vi "CTRE_Phoenix_TalonSRX_Open.vi"(6 "Invert":bool, 8 "error in":errorcluster, 10 "Device Number":u8) -> (0 "error out":errorcluster, 3 "CAN Talon SRX Ref":T1={"DeviceStatus"={"status"=FALSE, "code"=0, "source"=""}, "Type"=enum."PWM", "PWM"={"PWM Channel"=enum."PWM 1", "DeadBand"={"Name"="", "maxPositivePwm"=0, "minPositivePwm"=0, "centerPwm"=0, "maxNegativePwm"=0, "minNegativePwm"=0, "angularRange"=0}}, "CAN"={"Device Number"=0, "SetOutput VI Ref"=variant(enum8{"Percent VBus", "Current", "Speed", "Position", "Voltage"} enum."Percent VBus"), "GetOutput VI Ref"=variant(refnum<k1> refnum), "Enable VI Ref"=variant(dbl 12.0), "Disable VI Ref"=variant(enum8{"Percent VBus", "Speed", "Position", "Slave", "Unchanged / Invalid", "Voltage Compensation", "Current", "Motion Profile"} enum."Percent VBus"), "Data"=variant}, "Invert"=FALSE, "DIO PWM"={"PWM \"Enable\" Channel"=enum."Invalid", "DIOChannel"=enum."Invalid", "PWM Rate"=0.0}})   [LabVIEW 2020]
doc: "Creates a reference to the CAN-connected Talon SRX motor controller you specify. You must open a reference before using any other VIs on this palette. After you open a reference to the Talon SRX motor controller, you can use the other Talon SRX VIs to configure and control the Talon SRX. This reference is compatible with the WPI Robotics Motor VIs.\n\n<B>Control Mode</B> is the desired control mode of the Talon SRX.\n\n<B>Device Number</B> is the Talon SRX Device ID on the CAN bus.\n\n<B>Master Device Number</B> is the CAN bus Device ID of the master controller that this controller is to follow.\n\n<B>Invert</B> enables/disables inverting the motor when using the WPI Robotics SetOutput.vi."
uses:
  <vilib>/Rock Robotics/WPI/MotorControl/WPI_MotorControlDeviceRef.ctl
  <vilib>/Rock Robotics/WPI/MotorControl/WPI_MotorControlType.ctl
  <vilib>/Rock Robotics/SystemInterfaces/DIO/FPGA_DIOPWMChannel.ctl
  <vilib>/Rock Robotics/WPI/PWM/WPI_PWMDeadband.ctl
  <vilib>/Rock Robotics/SystemInterfaces/DIO/FPGA_DIOChannel.ctl
  <vilib>/Rock Robotics/WPI/ThirdParty/Phoenix-LabVIEW/Motor Controller/Controls/CTRE_Phoenix_MotorControl_DevRefData.ctl
  <vilib>/Rock Robotics/WPI/ThirdParty/Phoenix-LabVIEW/Motor Controller/Controls/CTRE_Phoenix_MotorControl_ControlMode.ctl
  <vilib>/Rock Robotics/WPI/ThirdParty/Phoenix-LabVIEW/Controls/DriverLib.ctl
  <vilib>/Rock Robotics/SystemInterfaces/NetworkCommunication/NetComm_UsageReport_ResourceType.ctl
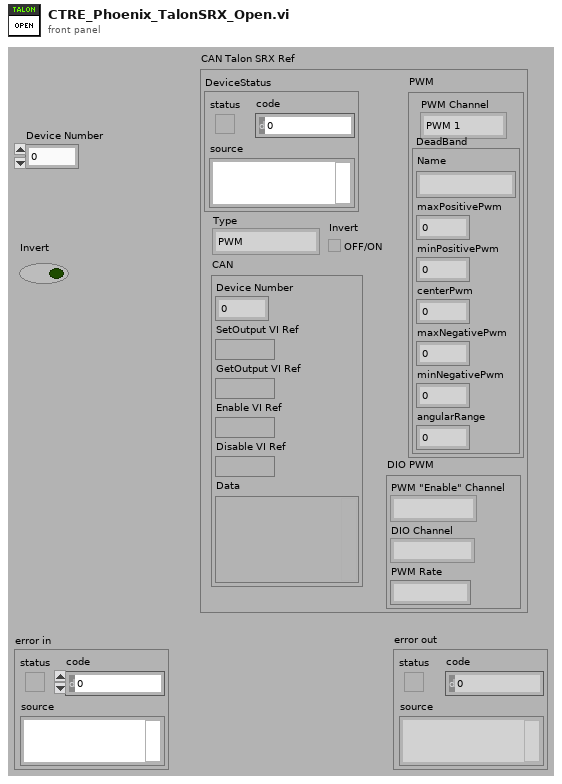
[diagram p1: front panel]
types:
  T1 = typedef "WPI_MotorControlDeviceRef.ctl" = cluster{"DeviceStatus":errorcluster, "Type":T2, "PWM":cluster{"PWM Channel":T3, "DeadBand":T4}, "CAN":cluster{"Device Number":u8, "SetOutput VI Ref":variant, "GetOutput VI Ref":variant, "Enable VI Ref":variant, "Disable VI Ref":variant, "Data":variant}, "Invert":bool, "DIO PWM":cluster{"PWM \"Enable\" Channel":T3, "DIOChannel":T5, "PWM Rate":dbl}}
  T2 = typedef "WPI_MotorControlType.ctl" = enum16{"PWM", "CAN", "DIO PWM"}
  T3 = typedef "FPGA_DIOPWMChannel.ctl" = enum8{"PWM 0", "PWM 1", "PWM 2", "PWM 3", "PWM 4", "PWM 5", "PWM 6", "PWM 7", "PWM 8", "PWM 9", "PWM MXP 0", "PWM MXP 1", "PWM MXP 2", "PWM MXP 3", "PWM MXP 4", "PWM MXP 5", "PWM MXP 6", "PWM MXP 7", "PWM MXP 8", "PWM MXP 9", "Invalid"}
  T4 = typedef "WPI_PWMDeadband.ctl" = cluster{"Name":string, "maxPositivePwm":i32, "minPositivePwm":i32, "centerPwm":i32, "maxNegativePwm":i32, "minNegativePwm":i32, "angularRange":u16}
  T5 = typedef "FPGA_DIOChannel.ctl" = enum8{"DIO 0", "DIO 1", "DIO 2", "DIO 3", "DIO 4", "DIO 5", "DIO 6", "DIO 7", "DIO 8", "DIO 9", "DIO MXP 0", "DIO MXP 1", "DIO MXP 2", "DIO MXP 3", "DIO MXP 4", "DIO MXP 5", "DIO MXP 6", "DIO MXP 7", "DIO MXP 8", "DIO MXP 9", "DIO MXP 10", "DIO MXP 11", "DIO MXP 12", "DIO MXP 13", "DIO MXP 14", "DIO MXP 15", "SPI Port CS1", "SPI Port CS2", "SPI Port CS3", "SPI Port MISO", "SPI Port MOSI", "Invalid"}
  T6 = typedef "CTRE_Phoenix_MotorControl_DevRefData.ctl" = cluster{"Library":path, "handle":u64, "Control Mode":T7, "UsageFrame":u32, "RefNumName":string, "arbID":u32}
  T7 = typedef "CTRE_Phoenix_MotorControl_ControlMode.ctl" = u16
  T8 = typedef "NetComm_UsageReport_ResourceType.ctl" = enum8{"Controller", "Module", "Language", "CANPlugin", "Accelerometer", "ADXL345", "AnalogChannel", "AnalogTrigger", "AnalogTriggerOutput", "CANJaguar", "Compressor", "Counter", "Dashboard", "DigitalInput", "DigitalOutput", "DriverStationCIO", "DriverStationEIO", "DriverStationLCD", "Encoder", "GearTooth", "Gyro", "I2C", "Framework", "Jaguar", "Joystick", "Kinect", "KinectStick", "PIDController", "Preferences", "PWM", "Relay", "RobotDrive", "SerialPort", "Servo", "Solenoid", "SPI", "Task", "Ultrasonic", "Victor", "Button", "Command", "AxisCamera", "PCVideoServer", "SmartDashboard", "Talon", "HiTechnicColorSensor", "HiTechnicAccel", "HiTechnicCompass", "SRF08", "AnalogOutput", "Victor SP", "Talon SRX", "CAN Talon SRX", "ADXL362 Accel", "ADXRS450 Gyro", "Rev SPARK", "Mindsensors SD540", "Digital Filter", "ADIS16448", "PDP", "PCM", "PigeonIMU", "Nidec Brushless", "CTRE CANifier", "CTRE TalonFX", "CTRE Future 1", "CTRE Future 2", "CTRE Future 3", "CTRE Future 4", "CTRE Future 5", "CTRE Future 6", "Linear Filter", "Xbox Controller", "USB Camera", "NavX", "Pixy", "Pixy2", "ScanseSweep", "Shuffleboard", "CAN", "Digilent DMC60", "PWM Victor SPX", "Rev SPARK MAX PWM", "Rev SPARK MAX CAN", "ADIS16470", "PIDController2", "ProfiledPIDController", "Kinematics", "Odometry", "Units", "Trapezoid Profile", "DutyCycle", "Addressable LEDs", "Fusion Venom"}
  T9 = typedef "DriverLib.ctl" = path
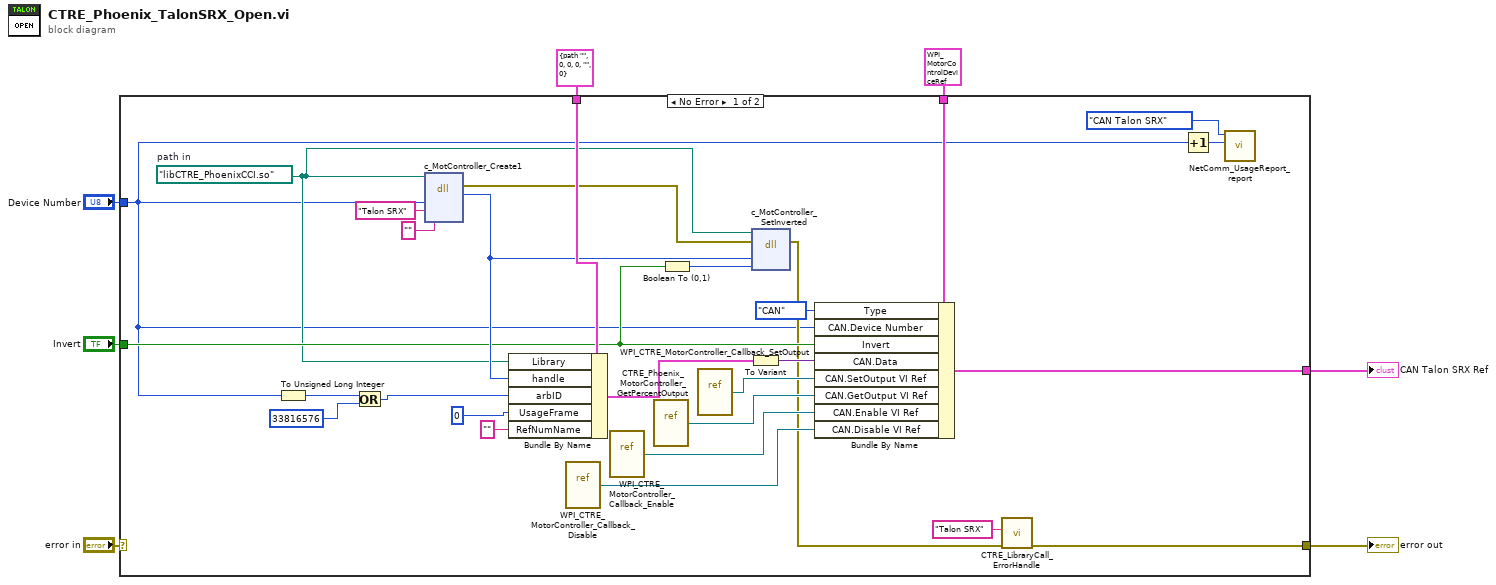
[diagram p0: block diagram]
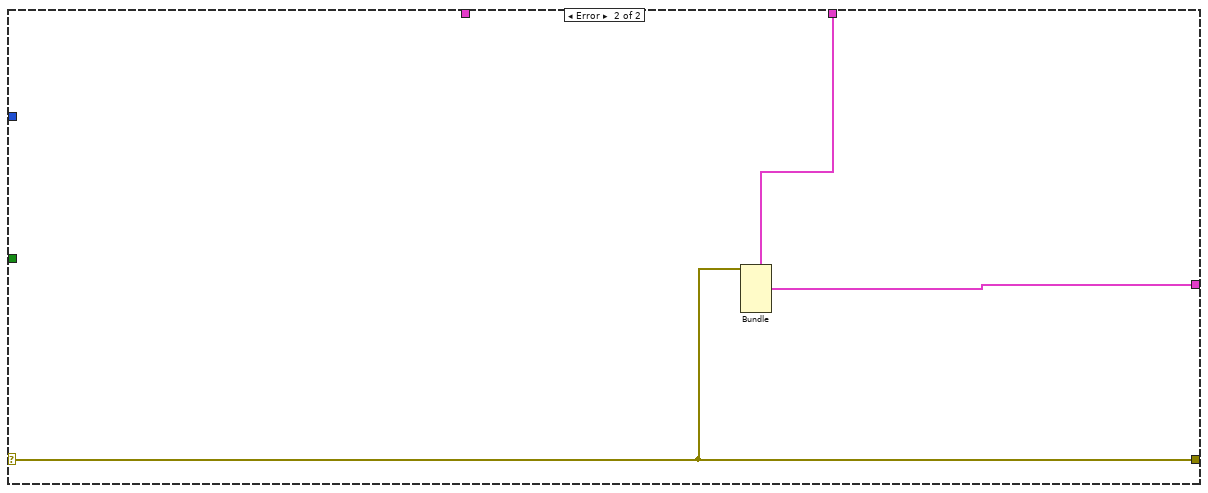
[diagram p2: hidden frame]
diagram:
  n1 = case shown="No Error" "error in" {
    selector: "error in" -> [_ w36]
    tunnel: [w14 w36] -> w7
    tunnel: "Invert" -> [w18 _]
    tunnel: T1 {"DeviceStatus"={"status"=FALSE, "code"=0, "source"=""}, "Type"=enum."CAN", "PWM"={"PWM Channel"=enum."PWM 1", "DeadBand"={"Name"="", "maxPositivePwm"=0, "minPositivePwm"=0, "centerPwm"=0, "maxNegativePwm"=0, "minNegativePwm"=0, "angularRange"=0}}, "CAN"={"Device Number"=0, "SetOutput VI Ref"=variant(refnum<vi> refnum), "GetOutput VI Ref"=variant(refnum<vi> refnum), "Enable VI Ref"=variant(refnum<vi> refnum), "Disable VI Ref"=variant(refnum<vi> refnum), "Data"=variant(cluster{"Control Mode":enum8{"Percent VBus", "Speed", "Position", "Slave", "Unchanged / Invalid", "Voltage Compensation", "Current", "Motion Profile"}, "Encoder Initial Position":dbl, "MaxVout":dbl} {"Control Mode"=enum."Percent VBus", "Encoder Initial Position"=0.0, "MaxVout"=12.0})}, "Invert"=FALSE, "DIO PWM"={"PWM \"Enable\" Channel"=enum."Invalid", "DIOChannel"=enum."Invalid", "PWM Rate"=0.0}} ("CAN Talon SRX Ref") -> [w35 w38]
    tunnel: "Device Number" -> [w10 _]
    tunnel: [w29 w37] -> w1
    tunnel: T6 {"Library"=path "", "handle"=0, "Control Mode"=0, "UsageFrame"=0, "RefNumName"="", "arbID"=0} -> [w26 _]
    frame No Error {
      w17 = T9 path "libCTRE_PhoenixCCI.so"  # path in
      n2 = To Unsigned Long Integer(number=w10) -> (unsigned 32bit integer=w22:u32)
      n3 = Or(x=w22, y=u32 33816576 ("baseID")) -> (x .or. y?=w21:u32)
      n4 = dll-call lib="?" fn="c_MotController_Create1"(path in=w17, "deviceID"=w10, "model"="Talon SRX", "canbus"="") -> (error out=w13:errorcluster, "return type"=w19:u64)  [unwired: 5 in, 1 out]
      n5 = Bundle By Name(cluster=w26, "Library"=w17, "handle"=w19, "arbID"=w21, "UsageFrame"=u32 0, "RefNumName"="") -> (w27:T6)
      n6 = vi-ref <vilib>:"WPI_CTRE_MotorController_Callback_Disable.vi"() -> (w30:refnum<vi>)
      n7 = vi-ref <vilib>:"WPI_CTRE_MotorController_Callback_Enable.vi"() -> (w31:refnum<vi>)
      n8 = vi-ref <vilib>:"CTRE_Phoenix_MotorController_GetPercentOutput.vi"() -> (w32:refnum<vi>)
      n9 = Boolean To (0,1)(Boolean=w18) -> (0, 1=w20:i16)
      n10 = vi-ref <vilib>:"WPI_CTRE_MotorController_Callback_SetOutput.vi"() -> (w33:refnum<vi>)
      n11 = To Variant(anything=w27) -> (Variant=w28:variant)
      n12 = dll-call lib="?" fn="c_MotController_SetInverted"(path in=w17, error in=w13, "handle"=w19, "Invert?"=w20) -> (error out=w16:errorcluster)  [unwired: 4 in, 1 out]
      n13 = Bundle By Name(cluster=w35, "Type"=WPI_MotorControlType."CAN", "CAN.Device Number"=w10, "Invert"=w18, "CAN.Data"=w28, "CAN.SetOutput VI Ref"=w33, "CAN.GetOutput VI Ref"=w32, "CAN.Enable VI Ref"=w31, "CAN.Disable VI Ref"=w30) -> (w29:T1)
      n14 = call <vilib>:"CTRE_LibraryCall_ErrorHandle.vi"("error in"=w16, "DeviceType"="Talon SRX") -> ("error out"=w14:errorcluster)  [unwired: 9 in]
      n15 = Increment(x=w10) -> (x+1=w12:u8)
      n16 = call <vilib>:"NetComm_UsageReport_report.vi"("Instance Number"=w12, "Resource Type"=NetComm_UsageReport_ResourceType."CAN Talon SRX") -> ()  [unwired: 10 in]
    }
    frame Error {
      n17 = Bundle(cluster=w38, "DeviceStatus"=w36) -> (w37:T1)  [unwired: 5 in]
    }
  }
  "CAN Talon SRX Ref" <- w1
  "error out" <- w7
